vi "LWXPS_Example_ElapsedTimeGet.vi"() -> ()   [LabVIEW 2013]
panel:
  out "Elapsed Time":dbl
  out "XPS Error String":string
  out "Error code":i32
  out "Error out":errorcluster caption="error out"
  in  "Instrument Key IN":string
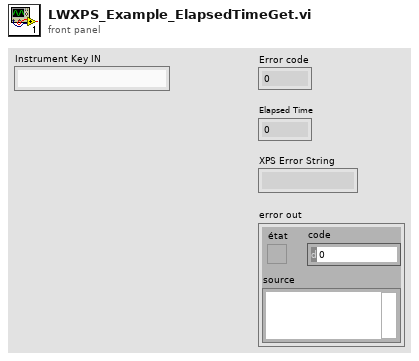
[diagram p1: front panel]
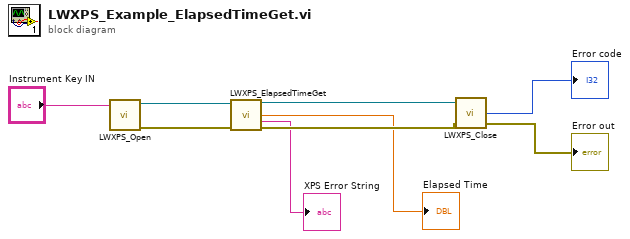
[diagram p0: block diagram]
diagram:
  n1 = call "LWXPS_Open.vi"("Instrument Key IN"="Instrument Key IN") -> ("error out"=w8:errorcluster, "CommandInterfaceXPS.XPS"=w9:refnum<k24>)  [unwired: 3 in, 2 out]
  n2 = call "LWXPS_ElapsedTimeGet.vi"("XPS Reference IN"=w9, "LabVIEW error IN"=w8) -> ("CommandInterfaceXPS.XPS"=w6:refnum<k24>, "Elapsed Time"=→"Elapsed Time":dbl, "XPS Error String"=→"XPS Error String":string, "LabVIEW error OUT"=w5:errorcluster)  [unwired: 9 in, 1 out]
  n3 = call "LWXPS_Close.vi"("error in (no error)"=w5, "XPS Reference"=w6) -> ("Error out"=→"Error out":errorcluster, "Error code"=→"Error code":i32)  [unwired: 2 in]
